vi "Enable Door.vi"(8 "error in (no error)":errorcluster, 10 "Disabled":T1(ring)=enum."Disabled", 11 "Abstract User Console in":refnum<class "Abstract User Console.lvclass">) -> (0 "error out":errorcluster, 3 "Abstract User Console out":refnum<class "Abstract User Console.lvclass">)   [LabVIEW 2019, in "Abstract User Console Actor.lvlib" / "Abstract User Console.lvclass"]
uses:
  Abstract User Console.lvclass
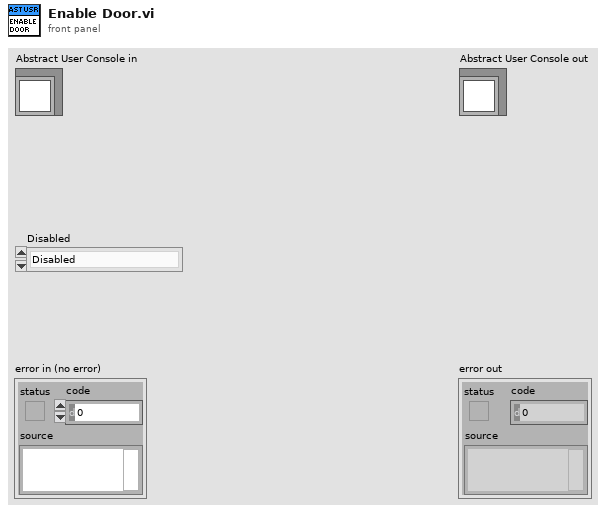
[diagram p1: front panel]
types:
  T1 = enum8{"Enabled", "Disabled", "Disabled and Grayed Out"}
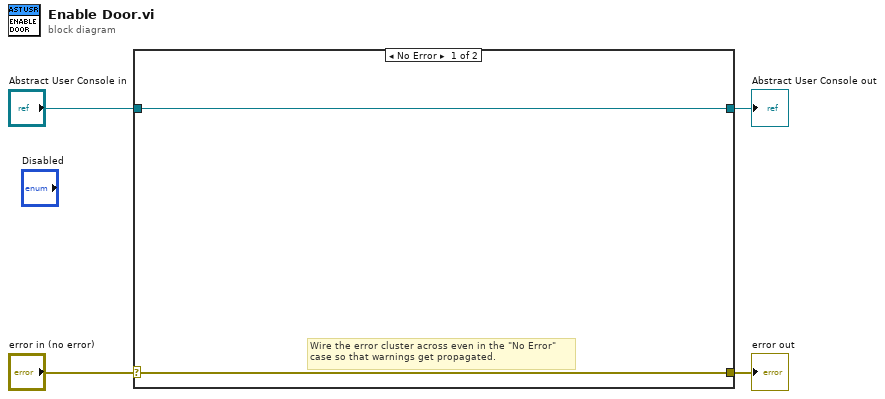
[diagram p0: block diagram]
diagram:
  n1 = case shown="No Error" "error in (no error)" {
    selector: "error in (no error)" -> [w5 w8]
    tunnel: [w5 w8] -> w3
    tunnel: [w6 w7] -> w1
    tunnel: "Abstract User Console in" -> [w6 w7]
    frame No Error {
      # "Wire the error cluster across even in the \"No Error\"\ncase so that warnings get propagated."
    }
    frame Error {
    }
  }
  "error out" <- w3
  "Abstract User Console out" <- w1
